vi "DeleteMeasurementFromDB.vi"(8 "error in (no error)":errorcluster, 10 "Measurement ID":string, 11 "DatabaseConnectionInfo":T1) -> (0 "error out":errorcluster)   [LabVIEW 2017]
uses:
  <vilib>/addons/database/Auxilliary.llb/DB Tools Transaction.ctl
  <vilib>/addons/database/Connection.llb/DB Tools Open Connec (Path).vi
  <vilib>/addons/database/Connection.llb/Conn Transaction.vi
  <vilib>/addons/database/NI_Database_API.lvlib
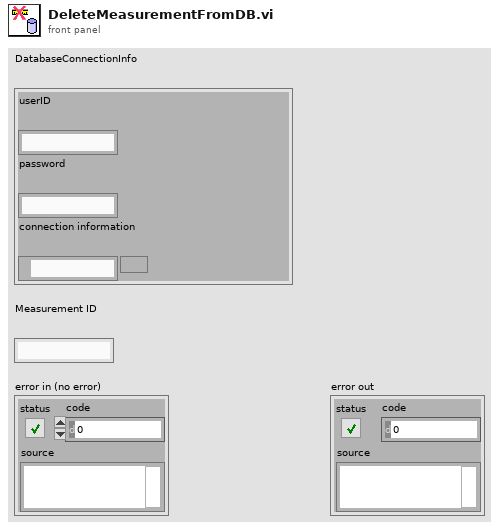
[diagram p1: front panel]
types:
  T1 = cluster{"userID":string, "password":string, "connection information":path}
  T2 = typedef "NI_Database_API.lvlib/DB Tools Transaction.ctl" = enum16{"begin", "commit", "rollback"}
  T3 = typedef "NI_Database_API.lvlib/Conn ObjectReference.ctl" = refnum<k1>
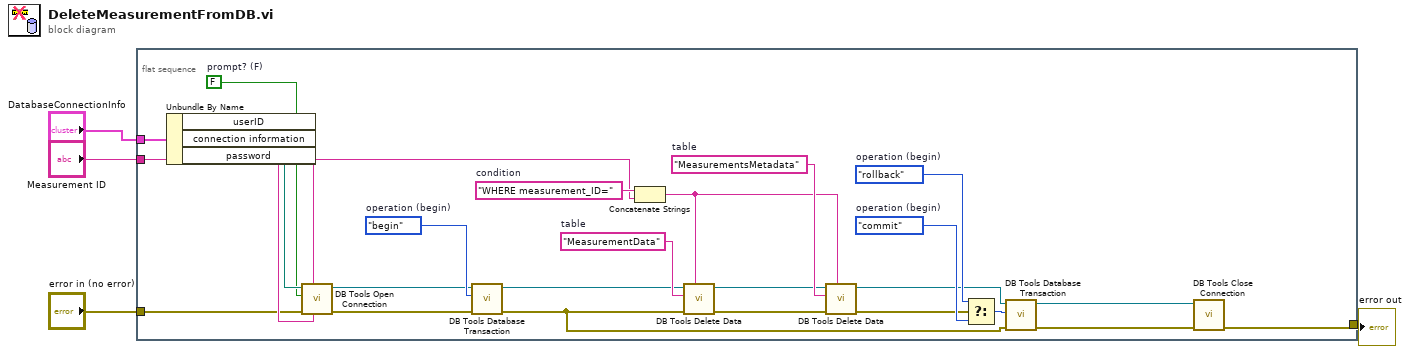
[diagram p0: block diagram]
diagram:
  n1 = flat-sequence {
    tunnel: [w24] -> w1
    tunnel: "DatabaseConnectionInfo" -> [w19]
    tunnel: "error in (no error)" -> [w18]
    tunnel: "Measurement ID" -> [w6]
    frame #0 {
      w12 = DB_Tools_Transaction."rollback"  # operation (begin)
      w11 = DB_Tools_Transaction."commit"  # operation (begin)
      w16 = DB_Tools_Transaction."begin"  # operation (begin)
      w20 = FALSE  # prompt? (F)
      w28 = "MeasurementsMetadata"  # table
      w29 = "MeasurementData"  # table
      w30 = "WHERE measurement_ID="  # condition
      n2 = Unbundle By Name(w19) -> ("userID"=w21:string, "connection information"=w23:path, "password"=w22:string)
      n3 = call-poly <vilib>:"DB Tools Open Connection.vi"("password"=w22, "userID"=w21, "error in (no error)"=w18, "prompt? (F)"=w20, "connection information"=w23) -> ("error out"=w14:errorcluster, "connection reference"=w15:T3)  [unwired: 3 in]
      n4 = call-poly <vilib>:"DB Tools Database Transaction.vi"("error in (no error)"=w14, "operation (begin)"=w16, "connection reference"=w15) -> ("error out"=w5:errorcluster, "connection reference out"=w13:T3)  [unwired: 3 in]
      n5 = Concatenate Strings(w30, w6) -> (w27:string)
      n6 = call <vilib>:"DB Tools Delete Data.vi"("condition"=w27, "error in (no error)"=w5, "table"=w29, "connection reference"=w13) -> ("error out"=w25:errorcluster, "connection reference out"=w26:T3)  [unwired: 6 in]
      n7 = call <vilib>:"DB Tools Delete Data.vi"("condition"=w27, "error in (no error)"=w25, "table"=w28, "connection reference"=w26) -> ("error out"=w9:errorcluster, "connection reference out"=w10:T3)  [unwired: 6 in]
      n8 = Select(t=w12, s=w9, f=w11) -> (s? t:f=w17:T2)
      n9 = call-poly <vilib>:"DB Tools Database Transaction.vi"("error in (no error)"=w5, "operation (begin)"=w17, "connection reference"=w10) -> ("error out"=w7:errorcluster, "connection reference out"=w8:T3)  [unwired: 3 in]
      n10 = call <vilib>:"DB Tools Close Connection.vi"("error in (no error)"=w7, "connection reference"=w8) -> ("error out"=w24:errorcluster)  [unwired: 5 in]
    }
  }
  "error out" <- w1
